vi "Image_Display[1].vi"() -> ()   [LabVIEW 2017]
panel:
  out "Image":T1(plugin-control)
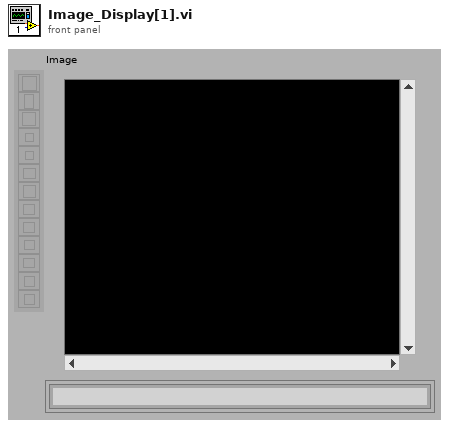
[diagram p1: front panel]
types:
  T1 = typedef "IMAQ Image.ctl" = refnum<image>
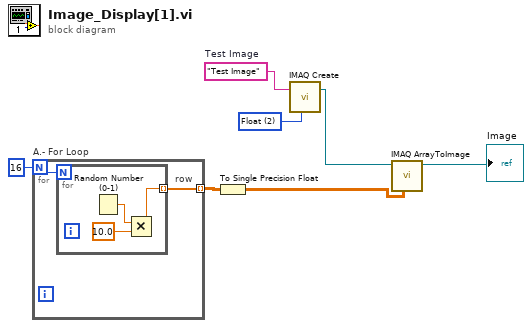
[diagram p0: block diagram]
diagram:
  w2 = u32 2 items=["8 bits", "16 bits", "Float", "Complex", "RGB", "HSL"] ("Image Type")
  w6 = "Test Image"  # Test Image
  n1 = for "A.- For Loop" {
    N: 16 -> [w9]
    tunnel: [w8] -> w3 mode=indexing
    # "row"
    n2 = for {
      N: w9 -> [_]
      tunnel: [w11] -> w8 mode=indexing
      n3 = Random Number (0-1)() -> (number: 0 to 1=w12:dbl)
      n4 = Multiply(x=w12, y=10.0) -> (x*y=w11:dbl)
    }
  }
  n5 = To Single Precision Float(number=w3) -> (single precision float=w1:sgl[][])
  n6 = call "IMAQ Create"("Image Name"=w6, "Image Type"=w2) -> ("New Image"=w7:T1)  [unwired: 3 in, 1 out]
  n7 = call "IMAQ ArrayToImage"("Image Pixels (Float)"=w1, "Image"=w7) -> ("Image Out"=→"Image":T1)  [unwired: 8 in, 1 out]
